vi "画结果.vi"(8 "error in (no error)":errorcluster, 9 "结果 2":T1(array[cluster]), 10 "结果":bool, 11 "处理后图像 In":T2(plugin-control)) -> (0 "error out":errorcluster, 3 "处理后图像 Out":T2(plugin-control))   [LabVIEW 2017]
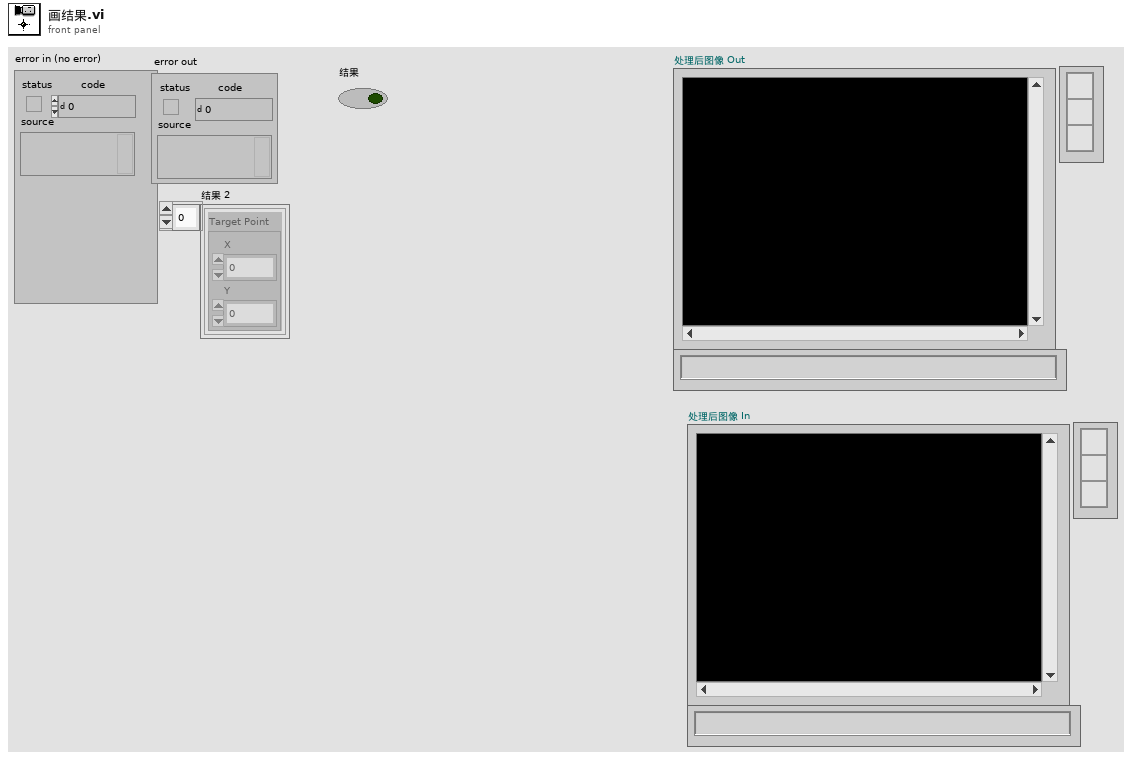
[diagram p1: front panel]
types:
  T1 = cluster{"Target Point":cluster{"X":dbl, "Y":dbl}}[]
  T2 = typedef "IMAQ Image.ctl" = refnum<image>
  T3 = cluster{"Desired Font (Application)":enum16{"User-specified Font", "Application Font", "System Font", "Dialog Font"}, "[User-specified Font]":cluster{"Font Name":string, "Size":i16, "Strikeout?":bool, "Italic?":bool, "Underline?":bool, "Outline?":bool, "Shadow?":bool, "Bold?":bool, "Rotation Angle":dbl}, "Horizontal Alignment":i16, "Vertical Alignment":i16}
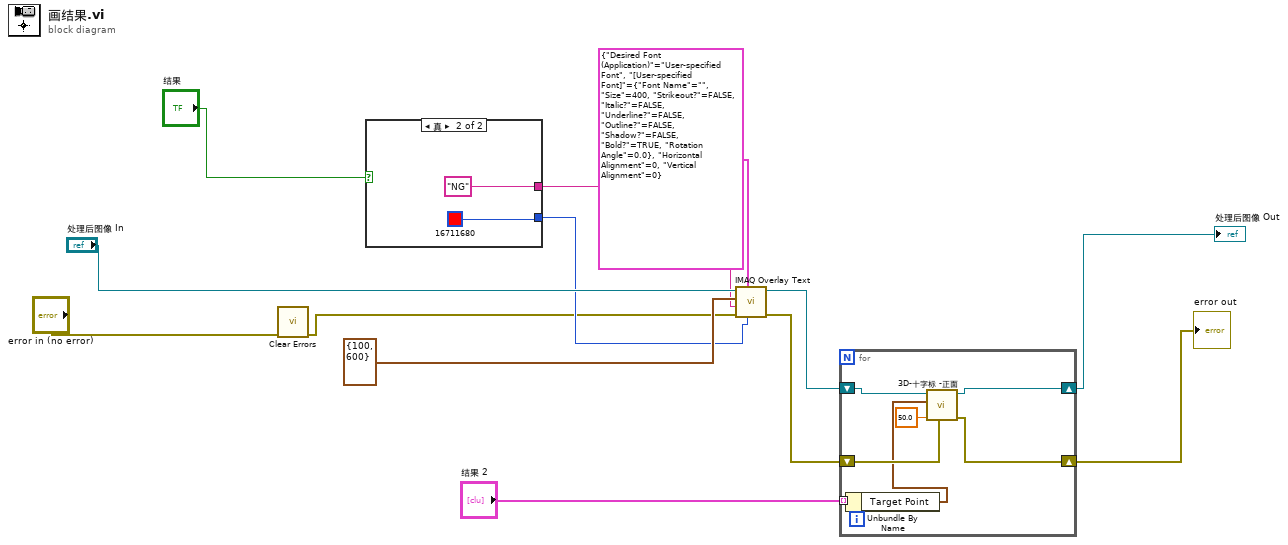
[diagram p0: block diagram]
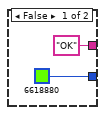
[diagram p2: hidden frame]
diagram:
  n1 = call <vilib>:"Clear Errors.vi"("error in (no error)"="error in (no error)") -> ("error out"=w6:errorcluster)  [unwired: 5 in, 1 out]
  n2 = case shown="真" "结果" {
    tunnel: ["OK" "NG"] -> w10
    tunnel: [u32 6618880 ("Text Color (black)") u32 16711680 ("Text Color (black)")] -> w8
    frame False {
    }
    frame True {
    }
  }
  n3 = call "IMAQ Overlay Text"("Text Color (black)"=w8, "Font, Size & Style"=T3 {"Desired Font (Application)"=enum."User-specified Font", "[User-specified Font]"={"Font Name"="", "Size"=400, "Strikeout?"=FALSE, "Italic?"=FALSE, "Underline?"=FALSE, "Outline?"=FALSE, "Shadow?"=FALSE, "Bold?"=TRUE, "Rotation Angle"=0.0}, "Horizontal Alignment"=0, "Vertical Alignment"=0}, "error in (no error)"=w6, "String"=w10, "Origin"=cluster{"X":i32, "Y":i32} {"X"=100, "Y"=600}, "Image"="处理后图像 In") -> ("error out"=w4:errorcluster, "Image Out"=w2:T2)  [unwired: 4 in]
  n4 = for {
    tunnel: "结果 2" -> [w19] mode=indexing
    shift-right: [w23] -> w1
    shift-left: w2 -> [w24]
    shift-right: [w21] -> w3
    shift-left: w4 -> [w22]
    n5 = Unbundle By Name(w19) -> ("Target Point"=w18:cluster{"X":dbl, "Y":dbl})
    n6 = call "3D-十字标 -正面.vi"("error in (no error)"=w22, "radius"=50.0, "Target Point"=w18, "输入图片"=w24) -> ("error out"=w21:errorcluster, "输出图片"=w23:T2)  [unwired: 6 in]
  }
  "处理后图像 Out" <- w1
  "error out" <- w3
